vi "Get Scan Software To Install.vi"(8 "error in (no error)":errorcluster, 10 "available software components":T1[](array[typedef]) {"component type" items=["standard", "hidden", "system", "unknown", "startup"]}) -> (0 "error out":errorcluster, 1 "found":bool, 2 "scan software to install":T1[](array[typedef]) {"component type" items=["standard", "hidden", "system", "unknown", "startup", "image"]})   [LabVIEW 2013]
uses:
  <vilib>/nisyscfg/Software 1.2.ctl
  <vilib>/nisyscfg/Component Type.ctl
  <vilib>/nisyscfg/nisyscfg.lvlib
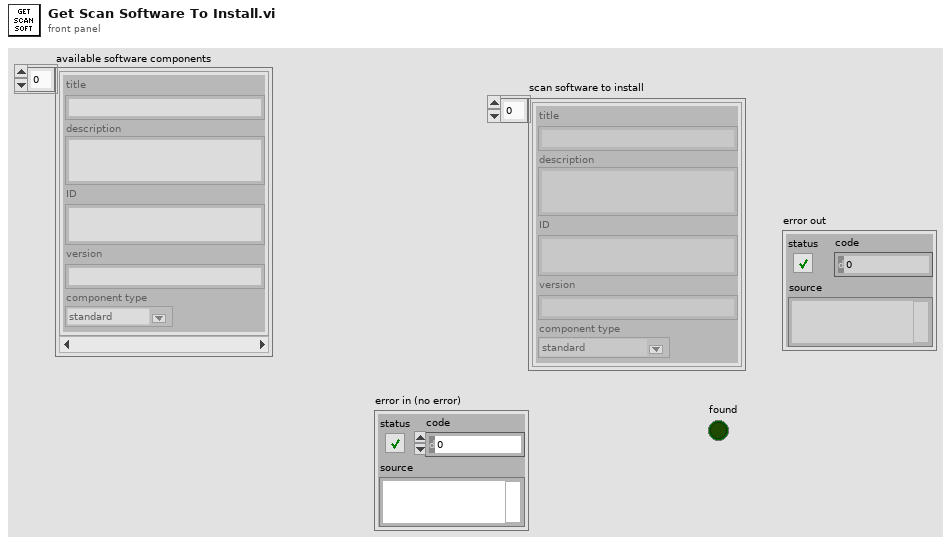
[diagram p1: front panel]
types:
  T1 = typedef "nisyscfg.lvlib/Software 1.2.ctl" = cluster{"title":string, "description":string, "ID":string, "version":string, "component type":T2}
  T2 = typedef "nisyscfg.lvlib/Component Type.ctl" = u32
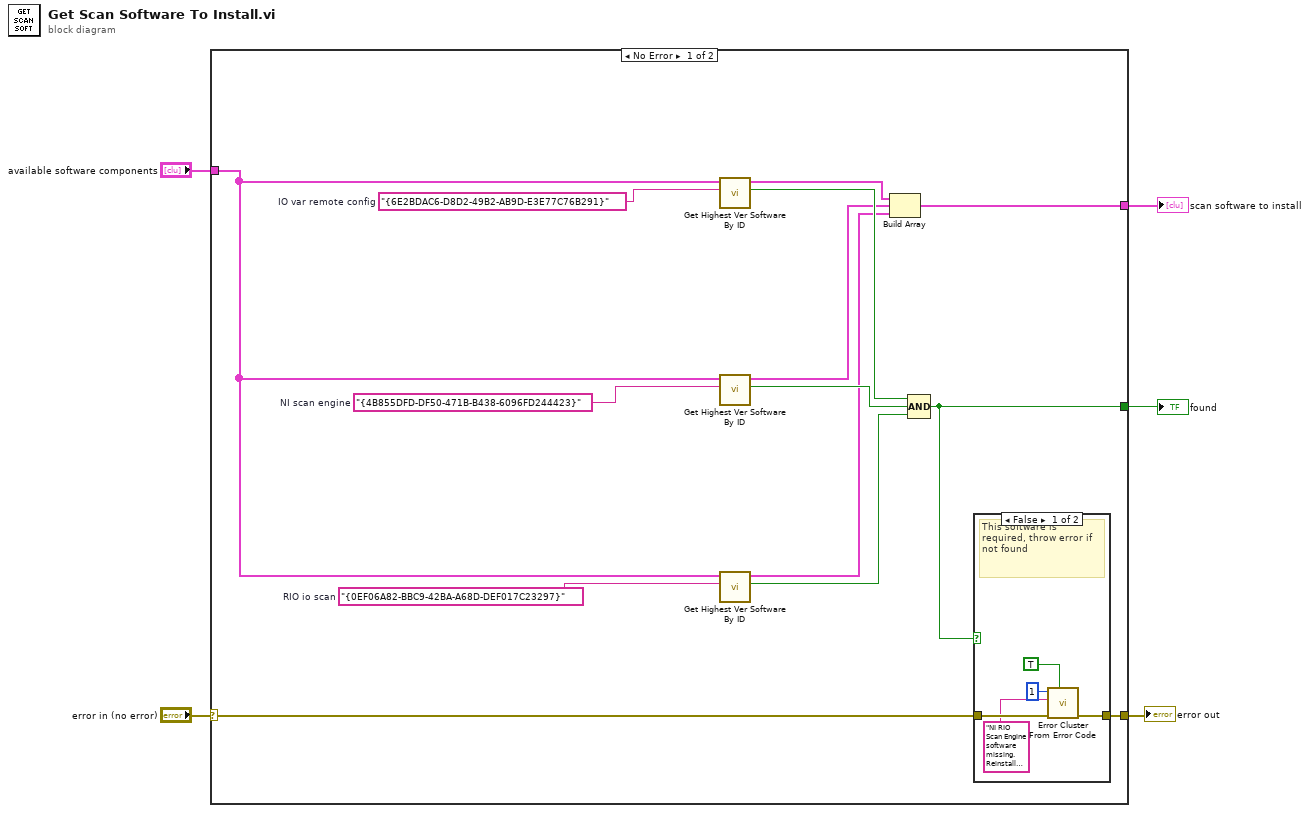
[diagram p0: block diagram]
diagram:
  n1 = case shown="No Error" "error in (no error)" {
    selector: "error in (no error)" -> [w17 w26]
    tunnel: "available software components" -> [w19 _]
    tunnel: [w18 _] -> w3
    tunnel: [w16 w26] -> w2
    tunnel: [w15 _] -> w1
    frame No Error {
      w6 = "{0EF06A82-BBC9-42BA-A68D-DEF017C23297}"  # RIO io scan
      w11 = "{4B855DFD-DF50-471B-B438-6096FD244423}"  # NI scan engine
      w12 = "{6E2BDAC6-D8D2-49B2-AB9D-E3E77C76B291}"  # IO var remote config
      n2 = call "Get Highest Ver Software By ID.vi"("ID"=w12, "available software components"=w19) -> ("found"=w14:bool, "Software"=w13:T1)  [unwired: 8 in]
      n3 = call "Get Highest Ver Software By ID.vi"("ID"=w11, "available software components"=w19) -> ("found"=w10:bool, "Software"=w9:T1)  [unwired: 8 in]
      n4 = call "Get Highest Ver Software By ID.vi"("ID"=w6, "available software components"=w19) -> ("found"=w7:bool, "Software"=w8:T1)  [unwired: 8 in]
      n5 = Build Array(w13, w9, w8) -> (w18:T1[])
      n6 = Compound Arithmetic op=AND(w14, w10, w7) -> (w15:bool)
      n7 = case shown="False" w15 {
        tunnel: w17 -> [w24 w25]
        tunnel: [w20 w25] -> w16
        frame False {
          # "This software is required, throw error if not found"
          n8 = call <vilib>:"Error Cluster From Error Code.vi"("show call chain? (False)"=TRUE, "error in (no error)"=w24, "error message (\"\")"="NI RIO Scan Engine software missing. Reinstall NI-RIO." ("error message (\"\")"), "error code (0)"=1) -> ("error out"=w20:errorcluster)  [unwired: 5 in]
        }
        frame True {
        }
      }
    }
    frame Error {
    }
  }
  "scan software to install" <- w3
  "error out" <- w2
  "found" <- w1
